vi "Read Configuration.vi"(8 "error in (no error)":errorcluster, 11 "ADAS PE Template in":refnum<class "ADAS PE Template.lvclass">) -> (0 "error out":errorcluster, 2 "Configuration":T1, 3 "ADAS PE Template out":refnum<class "ADAS PE Template.lvclass">)   [LabVIEW 2020, in "ADAS PE Template.lvlib" / "ADAS PE Template.lvclass"]
doc: "<b>Read Configuration</b>\nExtracts the configuration data from the Plugin class data."
uses:
  ADAS PE Template.lvclass
  Configuration.ctl
  ADAS PE Template.lvclass/ADAS PE Template.ctl
panel:
  # "#via_ignore"
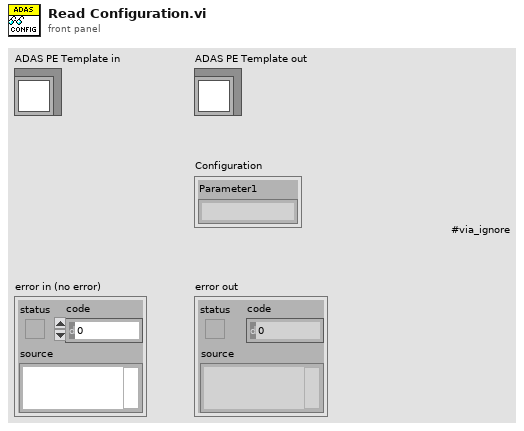
[diagram p1: front panel]
types:
  T1 = typedef "ADAS PE Template.lvlib/ADAS PE Template.lvclass/Configuration.ctl" = cluster{"Parameter1":string}
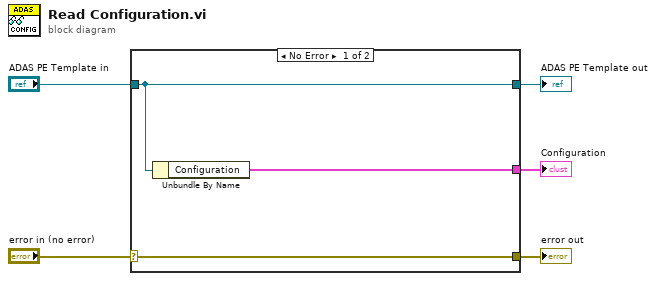
[diagram p0: block diagram]
diagram:
  n1 = case shown="No Error" "error in (no error)" {
    selector: "error in (no error)" -> [w8 w9]
    tunnel: [w8 w9] -> w4
    tunnel: [w7 w10] -> w2
    tunnel: "ADAS PE Template in" -> [w7 w10]
    tunnel: [w6 _] -> w1
    frame No Error {
      n2 = Unbundle By Name(w7) -> ("Configuration"=w6:T1)
    }
    frame Error {
    }
  }
  "error out" <- w4
  "ADAS PE Template out" <- w2
  "Configuration" <- w1
